vi "Main.vi"(8 "error in (no error)":errorcluster, 11 "StageSPIMBase in":refnum<class "StageSPIM.lvclass">) -> (0 "error out":errorcluster, 3 "component":refnum<class "StageSPIM.lvclass">)   [LabVIEW 2012, in "StageSPIM.lvclass"]
doc: "Main VI of the component."
uses:
  StageSPIM.lvclass
  <vilib>/Distrio/Murmex/Murmex/command_enum.ctl
  StageSPIM.lvclass/StageSPIM.ctl
  <vilib>/Distrio/Murmex/InitialiseMessage/InitialiseMessage.lvclass
  <vilib>/Distrio/Murmex/GenericMessage/GenericMessage.lvclass
  <vilib>/Distrio/Murmex/TerminateMessage/TerminateMessage.lvclass
  <vilib>/Distrio/Murmex/Murmex/update_cluster.ctl
  <vilib>/Distrio/Murmex/StopMessage/StopMessage.lvclass
  <vilib>/Distrio/Murmex/ConfigureMessage/ConfigureMessage.lvclass
  <vilib>/Distrio/Murmex/Murmex/Set configure at initialise.vi
  <vilib>/Distrio/Murmex/Murmex/Set log reference.vi
  <vilib>/Distrio/Murmex/Murmex/Set VI reference.vi
  <vilib>/Distrio/Murmex/Murmex/Get ID.vi
  <vilib>/Distrio/Murmex/Murmex/Set write log to disk.vi
  <vilib>/Distrio/Murmex/Murmex/Murmex.lvclass
  <vilib>/Distrio/Murmex/Message/Message.lvclass
panel:
  in  "Log position?":bool
  in  "button::stop":bool
  in  "button::configure":bool
  in  "button::quit":bool
  in  "Tab Control":enum32{"Main", "Debug"}(tab)
  in  "forwardFocus":bool
  in  "backFocus":bool
  in  "stepFocus":dbl[unit]
  out "currentFocus":dbl[unit]
  in  "speedFocus":dbl[unit]
  in  "targetFocus":dbl[unit]
  in  "forwardY":bool
  in  "backY":bool
  in  "stepY":dbl[unit]
  in  "forwardZ":bool
  in  "backZ":bool
  in  "stepZ":dbl[unit]
  in  "forwardX":bool
  in  "backX":bool
  in  "stepX":dbl[unit]
  in  "forwardA":bool
  in  "backA":bool
  in  "stepA":dbl[unit]
  out "currentA":dbl[unit]
  out "currentX":dbl[unit]
  out "currentY":dbl[unit]
  out "currentZ":dbl[unit]
  in  "speedZ":dbl[unit]
  in  "speedY":dbl[unit]
  in  "speedX":dbl[unit]
  in  "speedA":dbl[unit]
  in  "targetA":dbl[unit]
  in  "targetX":dbl[unit]
  in  "targetY":dbl[unit]
  in  "targetZ":dbl[unit]
  in  "button::send":bool
  out "log":string
  in  "command":T1
  in  "Generic command":string
  in  "ID":string="stage"
  out "terminate?":bool=TRUE
  # "Current\nposition"
  # "Target\nposition"
  # "Steps"
  # "Speed"
  # "A"
  # "X"
  # "Y"
  # "Z"
  # "Focus"
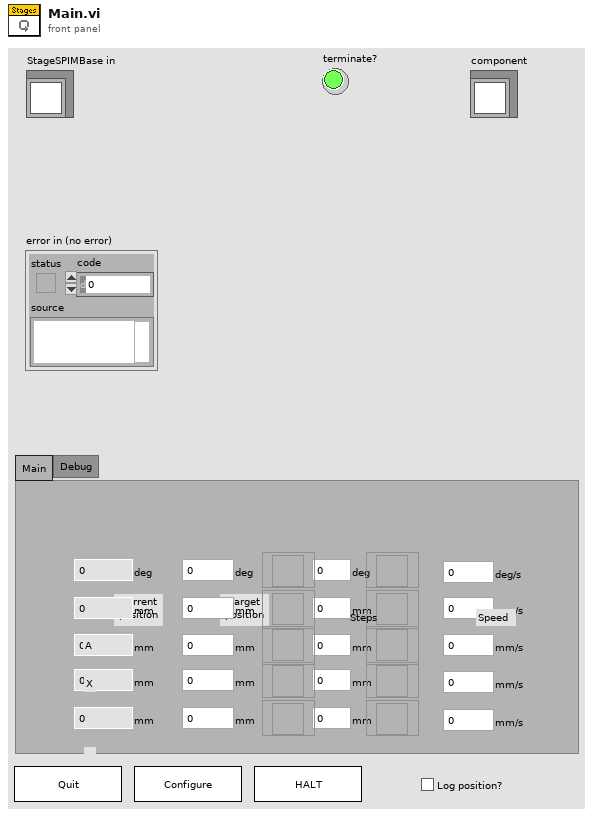
[diagram p1: front panel]
types:
  T1 = typedef "Murmex.lvlib/Murmex.lvclass/command_enum.ctl" = enum16{"null", "initialise", "reset", "terminate", "acknowledge", "update", "inspect", "inform", "proceed", "start", "stop", "fetch", "configure", "generic"}
  T2 = enum8{"Enabled", "Disabled", "Disabled and Grayed Out"}
  T3 = typedef "Murmex.lvlib/Murmex.lvclass/update_cluster.ctl" = cluster{"target ID":string, "key chains":string[], "values":variant[]}
  T4 = typedef "Murmex.lvlib/Murmex.lvclass/Event type enumerations.ctl" = enum16{"before", "after"}
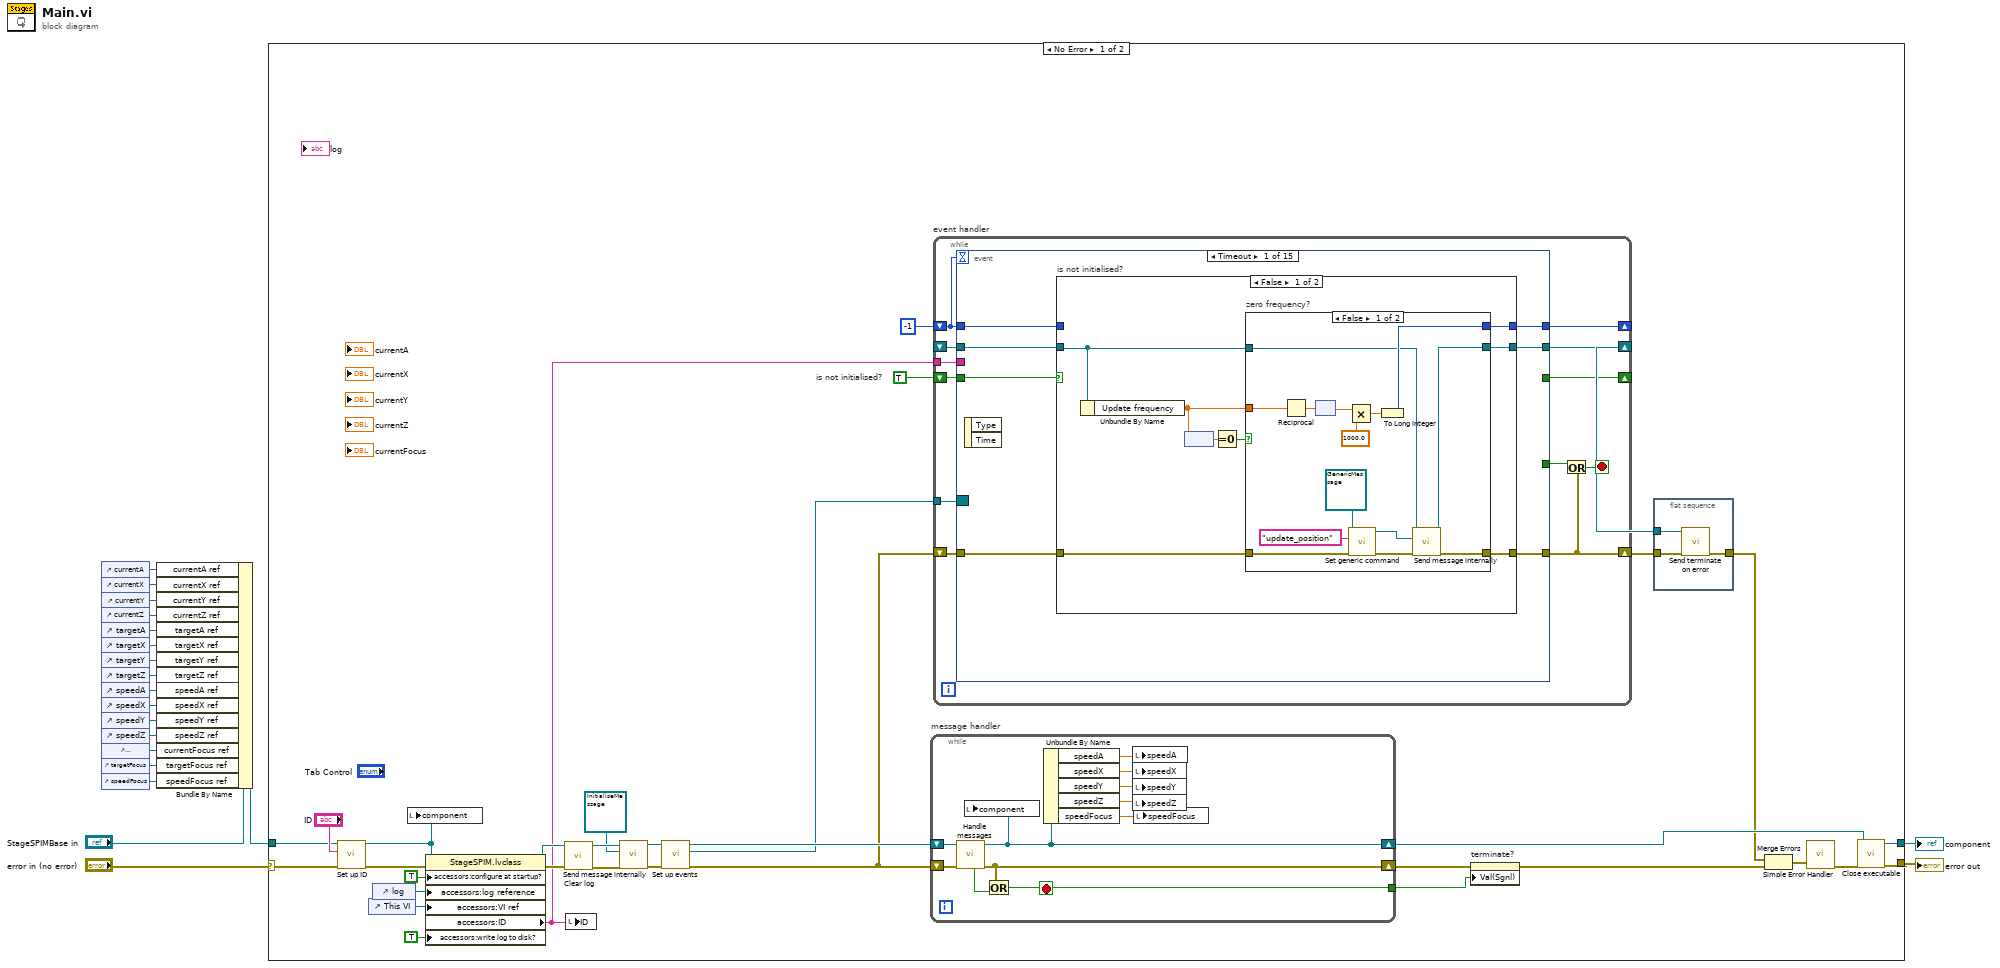
[diagram p0: block diagram]
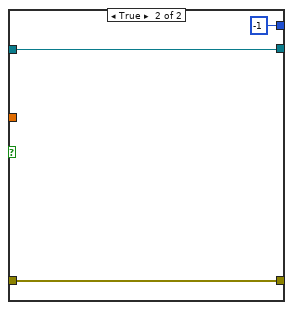
[diagram p2: hidden frame]
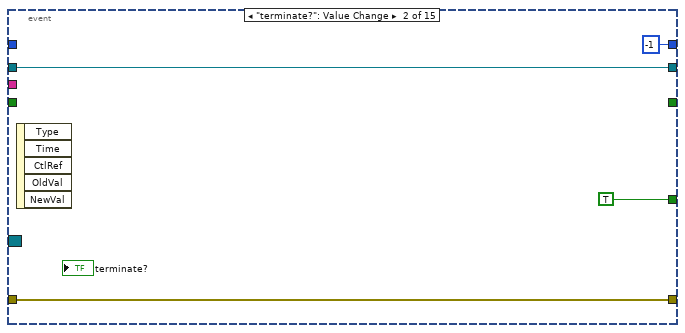
[diagram p4: hidden frame]
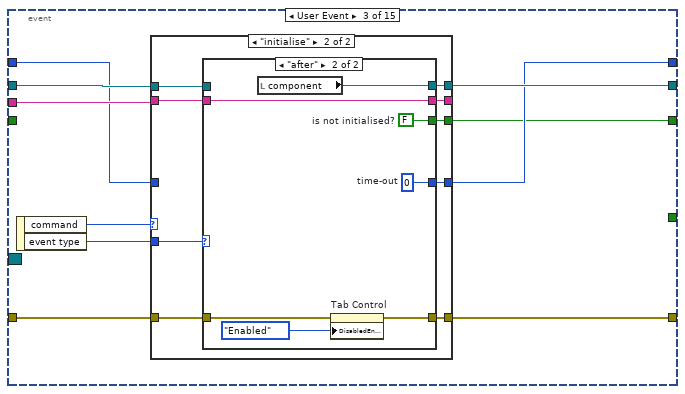
[diagram p5: hidden frame]
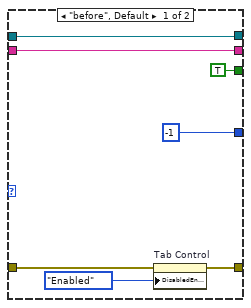
[diagram p7: hidden frame]
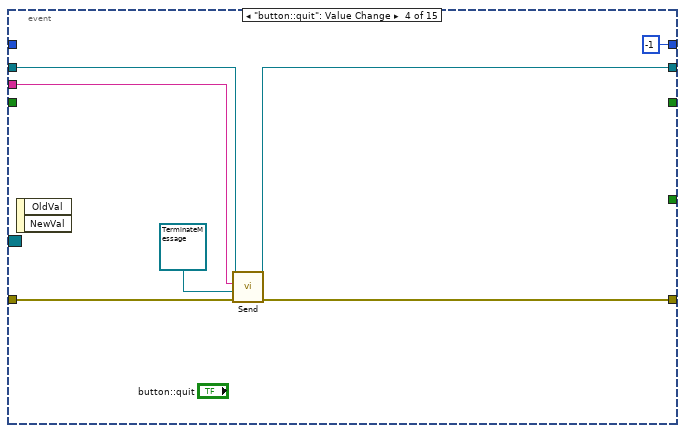
[diagram p8: hidden frame]
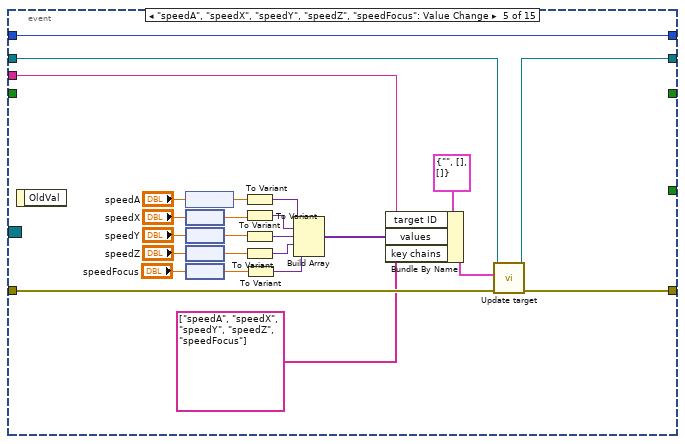
[diagram p9: hidden frame]
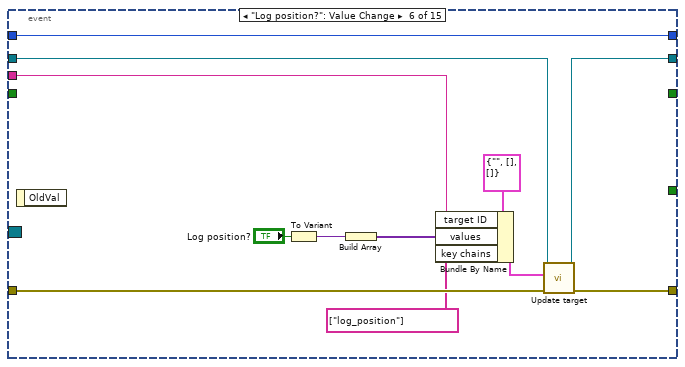
[diagram p10: hidden frame]
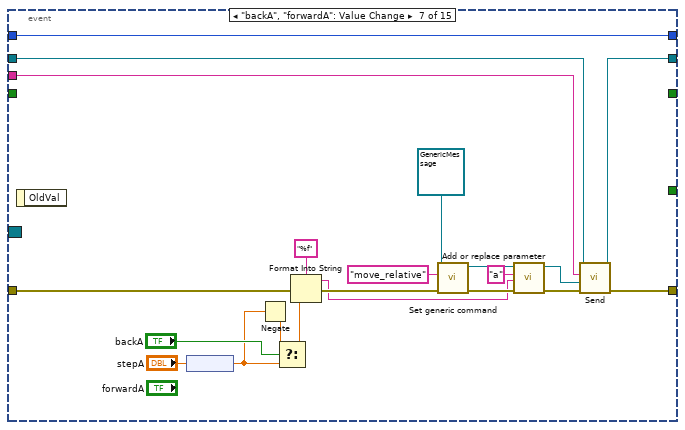
[diagram p11: hidden frame]
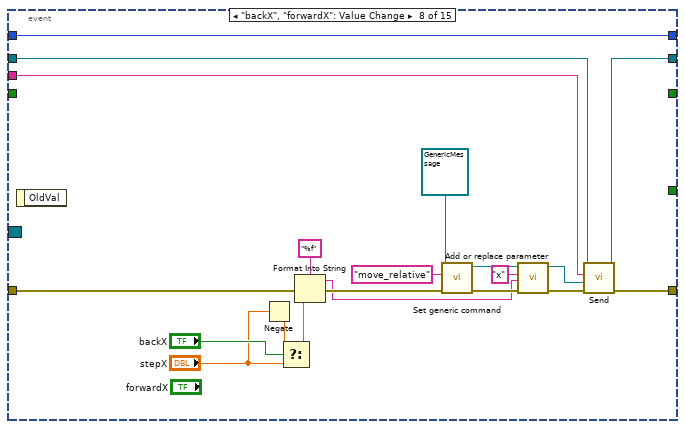
[diagram p12: hidden frame]
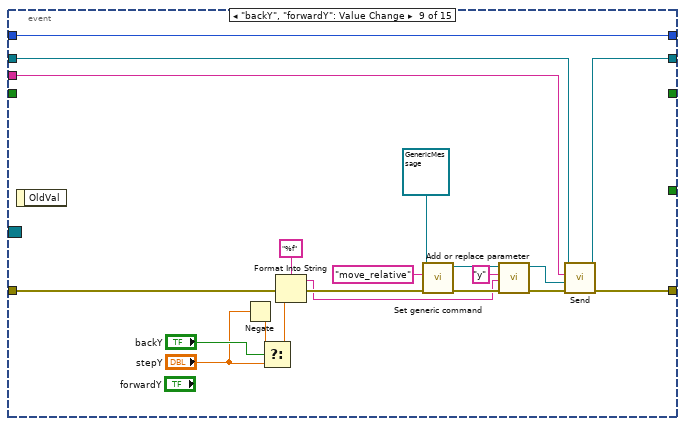
[diagram p13: hidden frame]
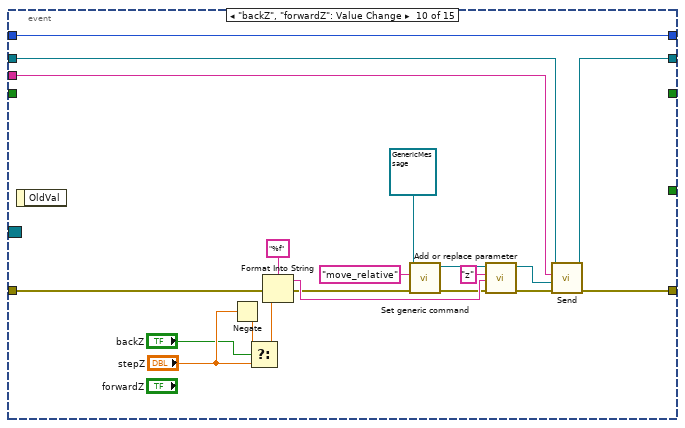
[diagram p14: hidden frame]
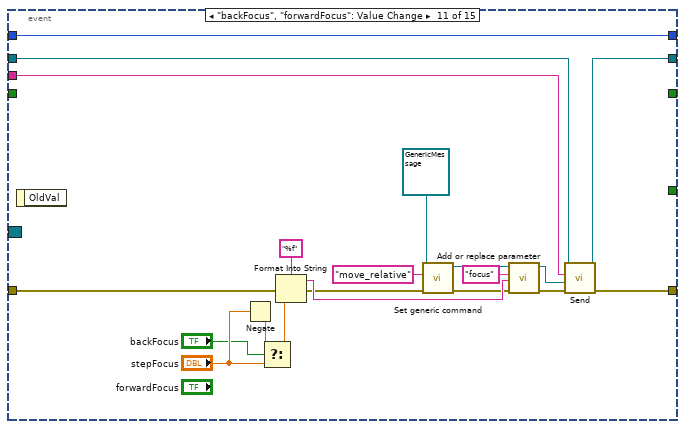
[diagram p15: hidden frame]
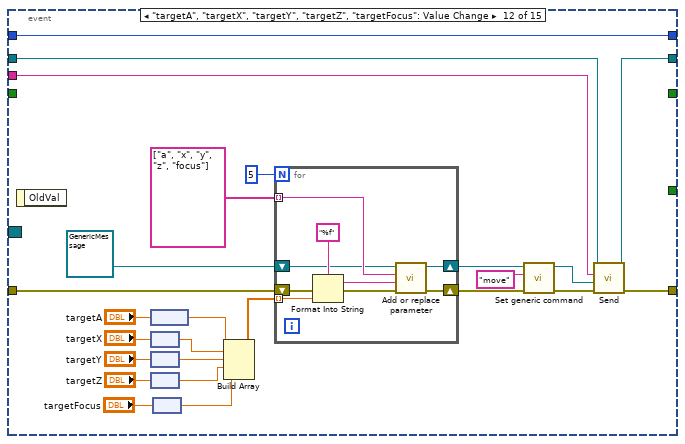
[diagram p16: hidden frame]
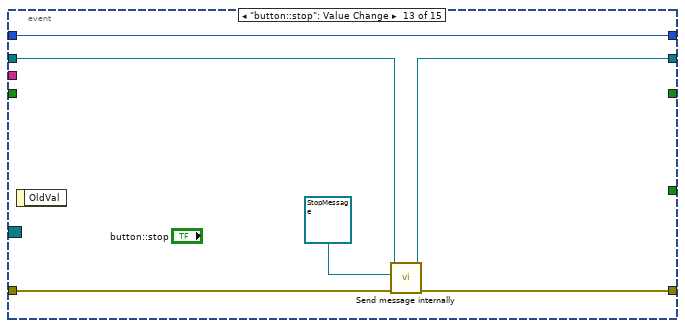
[diagram p17: hidden frame]
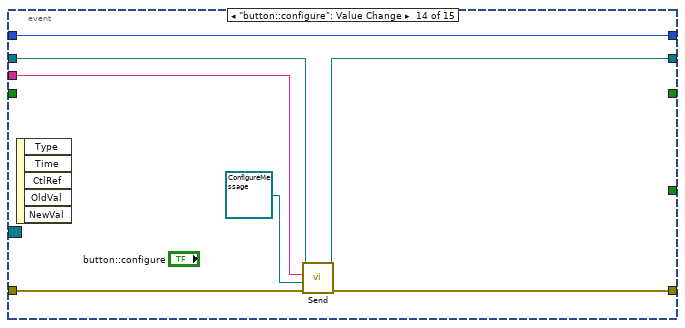
[diagram p18: hidden frame]
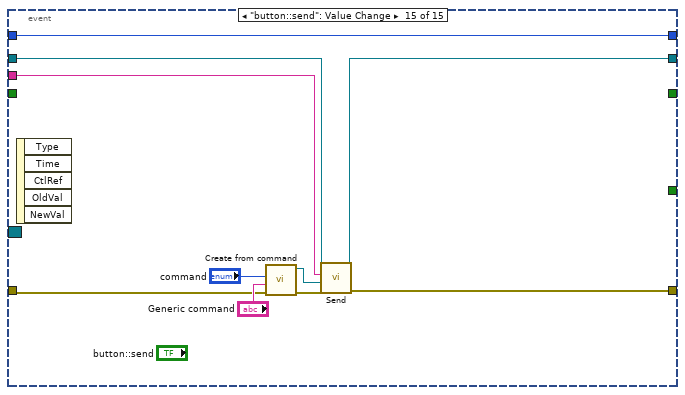
[diagram p19: hidden frame]
diagram:
  n1 = control-ref of="currentA"() -> (w15:refnum<vi>)
  n2 = control-ref of="currentX"() -> (w14:refnum<vi>)
  n3 = control-ref of="currentY"() -> (w13:refnum<vi>)
  n4 = control-ref of="currentZ"() -> (w12:refnum<vi>)
  n5 = control-ref of="targetA"() -> (w11:refnum<vi>)
  n6 = control-ref of="targetX"() -> (w10:refnum<vi>)
  n7 = control-ref of="targetY"() -> (w9:refnum<vi>)
  n8 = control-ref of="targetZ"() -> (w8:refnum<vi>)
  n9 = control-ref of="speedA"() -> (w7:refnum<vi>)
  n10 = control-ref of="speedX"() -> (w6:refnum<vi>)
  n11 = control-ref of="speedY"() -> (w5:refnum<vi>)
  n12 = control-ref of="speedZ"() -> (w4:refnum<vi>)
  n13 = control-ref of="currentFocus"() -> (w3:refnum<vi>)
  n14 = control-ref of="targetFocus"() -> (w2:refnum<vi>)
  n15 = control-ref of="speedFocus"() -> (w1:refnum<vi>)
  n16 = Bundle By Name(cluster="StageSPIMBase in", "currentA ref"=w15, "currentX ref"=w14, "currentY ref"=w13, "currentZ ref"=w12, "targetA ref"=w11, "targetX ref"=w10, "targetY ref"=w9, "targetZ ref"=w8, "speedA ref"=w7, "speedX ref"=w6, "speedY ref"=w5, "speedZ ref"=w4, "currentFocus ref"=w3, "targetFocus ref"=w2, "speedFocus ref"=w1) -> (w18:refnum<class "StageSPIM.lvclass">)
  n17 = case shown="No Error" "error in (no error)" {
    selector: "error in (no error)" -> [w52 w358]
    tunnel: w18 -> [w51 w359]
    tunnel: [w36 w358] -> w17
    tunnel: [w34 w359] -> w16
    frame No Error {
      w26 = TRUE  # is not initialised?
      n18 = call <vilib>:"Set up ID.vi"("error in (no error)"=w52, "component ID"="ID", "MurmexBase in"=w51) -> ("error out"=w50:errorcluster, "MurmexBase out"=w27:refnum<class "StageSPIM.lvclass">)  [unwired: 6 in, 1 out]
      n19 = control-ref of="This VI"() -> (w47:refnum<vi>)
      n20 = control-ref of="log"() -> (w48:refnum<vi>)
      n21 = local write "component"(w27) -> ()
      n22 = property class="StageSPIM.lvclass"(reference=w27, error in=w50, "accessors:configure at startup?"=TRUE ("configure at startup?"), "accessors:log reference"=w48, "accessors:VI ref"=w47, "accessors:write log to disk?"=TRUE ("write log to disk?")) -> (reference out=w45:refnum<class "StageSPIM.lvclass">, error out=w46:errorcluster, "accessors:ID"=w28:string)
      n23 = call <vilib>:"Clear log.vi"("error in (no error)"=w46, "MurmexBase in"=w45) -> ("error out"=w44:errorcluster, "MurmexBase out"=w43:refnum<class "StageSPIM.lvclass">)  [unwired: 8 in]
      n24 = local write "ID"(w28) -> ()
      n25 = call <vilib>:"Send message internally.vi"("error in (no error)"=w44, "Message"=refnum<class "InitialiseMessage.lvclass"> refnum ("Distrio Murmex 1.1:InitialiseMessage"), "Murmex in"=w43) -> ("error out"=w41:errorcluster, "Murmex out"=w40:refnum<class "StageSPIM.lvclass">)  [unwired: 7 in]
      n26 = call <vilib>:"Set up events.vi"("error in (no error)"=w41, "MurmexBase in"=w40) -> ("error out"=w33:errorcluster, "Event Registration Refnum"=w32:refnum<event-registration>, "MurmexBase out"=w39:refnum<class "StageSPIM.lvclass">)  [unwired: 7 in]
      n27 = while "message handler" {
        shift-right: [w355] -> w25
        shift-left: w33 -> [w357]
        shift-right: [w352] -> w35
        shift-left: w39 -> [w356]
        tunnel: [w353] -> w23
        stop <- w353 stop-if-true
        n28 = call <vilib>:"Handle messages.vi"("error in (no error)"=w357, "Murmex in"=w356) -> ("error out"=w355:errorcluster, "Murmex out"=w352:refnum<class "StageSPIM.lvclass">, "terminated?"=w354:bool)  [unwired: 7 in]
        n29 = local write "component"(w352) -> ()
        n30 = Or(x=w355, y=w354) -> (x .or. y?=w353:bool)
        n31 = Unbundle By Name(w352) -> ("speedA"=w351:dbl[unit], "speedX"=w350:dbl[unit], "speedY"=w349:dbl[unit], "speedZ"=w348:dbl[unit], "speedFocus"=w347:dbl[unit])
        n32 = local write "speedA"(w351) -> ()
        n33 = local write "speedX"(w350) -> ()
        n34 = local write "speedY"(w349) -> ()
        n35 = local write "speedZ"(w348) -> ()
        n36 = local write "speedFocus"(w347) -> ()
      }
      n37 = while "event handler" {
        shift-right: [w59] -> w30
        shift-left: w33 -> [w68]
        tunnel: w32 -> [w67]
        shift-right: [w65] -> _
        shift-left: -1 -> [w66]
        shift-right: [w62] -> w22
        shift-left: _ -> [w61]
        shift-right: [w57] -> _
        shift-left: w26 -> [w58]
        tunnel: w28 -> [w63]
        stop <- w64 stop-if-true
        n38 = event shown="[0] Timeout" {
          selector: w67 -> [_ _ _ _ _ _ _ _ _ _ _ _ _ _ _]
          dyn-events: _ -> [_ _ _ _ _ _ _ _ _ _ _ _ _ _ _]
          timeout: w66 -> [_ _ _ _ _ _ _ _ _ _ _ _ _ _ _]
          tunnel: w68 -> [w74 w107 w117 w150 w175 w185 w208 w211 w233 w253 w274 w293 w329 w336 w342]
          tunnel: w66 -> [w69 _ w109 _ w160 w182 w209 w210 w232 w254 w270 w309 w327 w330 w338]
          tunnel: [w75 -1 ("time-out") w110 -1 ("time-out") w160 w182 w209 w210 w232 w254 w270 w309 w327 w330 w338] -> w65
          tunnel: [w73 w107 w111 w149 w174 w186 w198 w217 w237 w256 w277 w313 w325 w335 w341] -> w59
          tunnel: w63 -> [_ _ w114 w146 w173 w181 w195 w214 w234 w255 w271 w310 _ w333 w337]
          tunnel: w61 -> [w71 w105 w113 w148 w172 w184 w197 w215 w235 w250 w273 w311 w328 w332 w340]
          tunnel: [w72 w105 w112 w147 w171 w183 w196 w216 w236 w257 w272 w312 w326 w331 w339] -> w62
          tunnel: [_ TRUE _ _ _ _ _ _ _ _ _ _ _ _ _] -> w60
          tunnel: w58 -> [w70 _ _ _ _ _ _ _ _ _ _ _ _ _ _]
          tunnel: [_ _ w108 _ _ _ _ _ _ _ _ _ _ _ _] -> w57
          event Timeout {
            n39 = event-data() -> ()  [unwired: 1 in, 2 out]
            n40 = case "is not initialised?" shown="False" w70 {
              tunnel: [w83 w101] -> w75
              tunnel: w74 -> [w82 w103]
              tunnel: [w81 w103] -> w73
              tunnel: [w80 w102] -> w72
              tunnel: w71 -> [w76 w102]
              tunnel: w69 -> [_ w101]
              frame False {
                n41 = Unbundle By Name(w76) -> ("Update frequency"=w79:dbl[unit])
                n42 = node(w79) -> (w78:dbl)
                n43 = Equal To 0?(x=w78) -> (x = 0?=w77:bool)
                n44 = case "zero frequency?" shown="False" w77 {
                  tunnel: [w93 -1] -> w83
                  tunnel: w82 -> [w85 w99]
                  tunnel: [w86 w99] -> w81
                  tunnel: w76 -> [w91 w100]
                  tunnel: [w84 w100] -> w80
                  tunnel: w79 -> [w92 _]
                  frame False {
                    n45 = Reciprocal(x=w92) -> (1/x=w97:dbl[unit])
                    n46 = node(w97) -> (w95:dbl)
                    n47 = Multiply(x=w95, y=1000.0) -> (x*y=w94:dbl)
                    n48 = call <vilib>:"Set generic command.vi"("error in (no error)"=w85, "generic command"="update_position", "GenericMessage in"=refnum<class "GenericMessage.lvclass"> refnum ("Message in")) -> ("error out"=w87:errorcluster, "GenericMessage out"=w88:refnum<class "GenericMessage.lvclass">)  [unwired: 7 in]
                    n49 = To Long Integer(number=w94) -> (32bit integer=w93:i32)
                    n50 = call <vilib>:"Send message internally.vi"("error in (no error)"=w87, "Message"=w88, "Murmex in"=w91) -> ("error out"=w86:errorcluster, "Murmex out"=w84:refnum<class "StageSPIM.lvclass">)  [unwired: 7 in]
                  }
                  frame True {
                  }
                }
              }
              frame True {
              }
            }
          }
          event "terminate?": Value Change {
            n51 = event-data() -> ()  [unwired: 1 in, 5 out]
          }
          event User Event {
            n52 = event-data() -> ("command"=w116:T1, "event type"=w115:T4)  [unwired: 1 in]
            n53 = case shown="\"initialise\"" w116 {
              tunnel: w117 -> [w119 w130]
              tunnel: [w119 w129] -> w111
              tunnel: w114 -> [w121 w128]
              tunnel: [w120 w127] -> w112
              tunnel: w113 -> [w120 w126]
              tunnel: [w121 w125] -> _
              tunnel: w115 -> [_ w124]
              tunnel: [w118 w123] -> w110
              tunnel: w109 -> [w118 _]
              tunnel: [_ w122] -> w108
              frame "null", Default {
              }
              frame "initialise" {
                n54 = case shown="\"after\"" w124 {
                  tunnel: [w136 w143] -> w129
                  tunnel: w130 -> [w137 w144]
                  tunnel: w128 -> [w134 w140]
                  tunnel: [w133 w142] -> w127
                  tunnel: w126 -> [w133 _]
                  tunnel: [w134 w140] -> w125
                  tunnel: [-1 w139] -> w123
                  tunnel: [TRUE ("is not initialised?") w138] -> w122
                  frame "before", Default {
                    n55 = property on="Tab Control" class="TabCtl (strict)"(error in=w137, "DisabledEnum"=T2."Enabled" ("Disabled")) -> (error out=w136:errorcluster)  [unwired: 1 in, 1 out]
                  }
                  frame "after" {
                    w138 = FALSE  # is not initialised?
                    w139 = 0  # time-out
                    n56 = local read "component"() -> (w142:refnum<class "StageSPIM.lvclass">)
                    n57 = property on="Tab Control" class="TabCtl (strict)"(error in=w144, "DisabledEnum"=T2."Enabled" ("Disabled")) -> (error out=w143:errorcluster)  [unwired: 1 in, 1 out]
                  }
                }
              }
            }
          }
          event "button::quit": Value Change {
            n58 = event-data() -> ()  [unwired: 1 in, 2 out]
            n59 = call <vilib>:"Send.vi"("error in (no error)"=w150, "Message"=refnum<class "TerminateMessage.lvclass"> refnum ("Murmex.lvlib:TerminateMessage"), "recipient"=w146, "Murmex in"=w148) -> ("error out"=w149:errorcluster, "Murmex out"=w147:refnum<class "StageSPIM.lvclass">)  [unwired: 6 in]
          }
          event "speedA", "speedX", "speedY", "speedZ", "speedFocus": Value Change {
            n60 = event-data() -> ()  [unwired: 1 in, 1 out]
            n61 = node("speedA") -> (w159:dbl)
            n62 = node("speedX") -> (w156:dbl)
            n63 = node("speedY") -> (w157:dbl)
            n64 = node("speedZ") -> (w158:dbl)
            n65 = node("speedFocus") -> (w154:dbl)
            n66 = To Variant(anything=w159) -> (Variant=w166:variant)
            n67 = To Variant(anything=w156) -> (Variant=w165:variant)
            n68 = To Variant(anything=w157) -> (Variant=w164:variant)
            n69 = To Variant(anything=w158) -> (Variant=w163:variant)
            n70 = To Variant(anything=w154) -> (Variant=w153:variant)
            n71 = Build Array(w166, w165, w164, w163, w153) -> (w162:variant[])
            n72 = Bundle By Name(cluster=T3 {"target ID"="", "key chains"=[], "values"=[]} ("update cluster"), "target ID"=w173, "values"=w162, "key chains"=string[] ["speedA", "speedX", "speedY", "speedZ", "speedFocus"]) -> (w152:T3)
            n73 = call <vilib>:"Update target.vi"("error in (no error)"=w175, "update cluster"=w152, "MurmexBase in"=w172) -> ("error out"=w174:errorcluster, "MurmexBase out"=w171:refnum<class "StageSPIM.lvclass">)  [unwired: 7 in]
          }
          event "Log position?": Value Change {
            n74 = event-data() -> ()  [unwired: 1 in, 1 out]
            n75 = To Variant(anything="Log position?") -> (Variant=w179:variant)
            n76 = Build Array(w179) -> (w178:variant[])
            n77 = Bundle By Name(cluster=T3 {"target ID"="", "key chains"=[], "values"=[]} ("update cluster"), "target ID"=w181, "values"=w178, "key chains"=string[] ["log_position"]) -> (w187:T3)
            n78 = call <vilib>:"Update target.vi"("error in (no error)"=w185, "update cluster"=w187, "MurmexBase in"=w184) -> ("error out"=w186:errorcluster, "MurmexBase out"=w183:refnum<class "StageSPIM.lvclass">)  [unwired: 7 in]
          }
          event "backA", "forwardA": Value Change {
            n79 = event-data() -> ()  [unwired: 1 in, 1 out]
            n80 = node("stepA") -> (w189:dbl)
            n81 = Negate(x=w189) -> (-x=w202:dbl)
            n82 = Select(t=w202, s="backA", f=w189) -> (s? t:f=w191:dbl)
            n83 = Format Into String(format string="%f", error in=w208, w191) -> (resulting string=w192:string, error out=w199:errorcluster)  [unwired: 1 in]
            n84 = call <vilib>:"Set generic command.vi"("error in (no error)"=w199, "generic command"="move_relative", "GenericMessage in"=refnum<class "GenericMessage.lvclass"> refnum ("Distrio Murmex 1.1:GenericMessage")) -> ("error out"=w206:errorcluster, "GenericMessage out"=w204:refnum<class "GenericMessage.lvclass">)  [unwired: 7 in]
            n85 = call <vilib>:"Add or replace parameter.vi"("error in (no error)"=w206, "value"=w192, "name"="a", "Message in"=w204) -> ("error out"=w205:errorcluster, "Message out"=w193:refnum<class "GenericMessage.lvclass">)  [unwired: 6 in]
            n86 = call <vilib>:"Send.vi"("error in (no error)"=w205, "Message"=w193, "recipient"=w195, "Murmex in"=w197) -> ("error out"=w198:errorcluster, "Murmex out"=w196:refnum<class "StageSPIM.lvclass">)  [unwired: 6 in]
          }
          event "backX", "forwardX": Value Change {
            n87 = event-data() -> ()  [unwired: 1 in, 1 out]
            n88 = Negate(x="stepX") -> (-x=w224:dbl[unit])
            n89 = Select(t=w224, s="backX", f="stepX") -> (s? t:f=w219:dbl[unit])
            n90 = Format Into String(format string="%f", error in=w211, w219) -> (resulting string=w220:string, error out=w223:errorcluster)  [unwired: 1 in]
            n91 = call <vilib>:"Set generic command.vi"("error in (no error)"=w223, "generic command"="move_relative", "GenericMessage in"=refnum<class "GenericMessage.lvclass"> refnum ("Distrio Murmex 1.1:GenericMessage")) -> ("error out"=w228:errorcluster, "GenericMessage out"=w226:refnum<class "GenericMessage.lvclass">)  [unwired: 7 in]
            n92 = call <vilib>:"Add or replace parameter.vi"("error in (no error)"=w228, "value"=w220, "name"="x", "Message in"=w226) -> ("error out"=w227:errorcluster, "Message out"=w221:refnum<class "GenericMessage.lvclass">)  [unwired: 6 in]
            n93 = call <vilib>:"Send.vi"("error in (no error)"=w227, "Message"=w221, "recipient"=w214, "Murmex in"=w215) -> ("error out"=w217:errorcluster, "Murmex out"=w216:refnum<class "StageSPIM.lvclass">)  [unwired: 6 in]
          }
          event "backY", "forwardY": Value Change {
            n94 = event-data() -> ()  [unwired: 1 in, 1 out]
            n95 = Negate(x="stepY") -> (-x=w244:dbl[unit])
            n96 = Select(t=w244, s="backY", f="stepY") -> (s? t:f=w239:dbl[unit])
            n97 = Format Into String(format string="%f", error in=w233, w239) -> (resulting string=w240:string, error out=w243:errorcluster)  [unwired: 1 in]
            n98 = call <vilib>:"Set generic command.vi"("error in (no error)"=w243, "generic command"="move_relative", "GenericMessage in"=refnum<class "GenericMessage.lvclass"> refnum ("Distrio Murmex 1.1:GenericMessage")) -> ("error out"=w248:errorcluster, "GenericMessage out"=w246:refnum<class "GenericMessage.lvclass">)  [unwired: 7 in]
            n99 = call <vilib>:"Add or replace parameter.vi"("error in (no error)"=w248, "value"=w240, "name"="y", "Message in"=w246) -> ("error out"=w247:errorcluster, "Message out"=w241:refnum<class "GenericMessage.lvclass">)  [unwired: 6 in]
            n100 = call <vilib>:"Send.vi"("error in (no error)"=w247, "Message"=w241, "recipient"=w234, "Murmex in"=w235) -> ("error out"=w237:errorcluster, "Murmex out"=w236:refnum<class "StageSPIM.lvclass">)  [unwired: 6 in]
          }
          event "backZ", "forwardZ": Value Change {
            n101 = event-data() -> ()  [unwired: 1 in, 1 out]
            n102 = Negate(x="stepZ") -> (-x=w263:dbl[unit])
            n103 = Select(t=w263, s="backZ", f="stepZ") -> (s? t:f=w268:dbl[unit])
            n104 = Format Into String(format string="%f", error in=w253, w268) -> (resulting string=w267:string, error out=w264:errorcluster)  [unwired: 1 in]
            n105 = call <vilib>:"Set generic command.vi"("error in (no error)"=w264, "generic command"="move_relative", "GenericMessage in"=refnum<class "GenericMessage.lvclass"> refnum ("Distrio Murmex 1.1:GenericMessage")) -> ("error out"=w259:errorcluster, "GenericMessage out"=w261:refnum<class "GenericMessage.lvclass">)  [unwired: 7 in]
            n106 = call <vilib>:"Add or replace parameter.vi"("error in (no error)"=w259, "value"=w267, "name"="z", "Message in"=w261) -> ("error out"=w260:errorcluster, "Message out"=w266:refnum<class "GenericMessage.lvclass">)  [unwired: 6 in]
            n107 = call <vilib>:"Send.vi"("error in (no error)"=w260, "Message"=w266, "recipient"=w255, "Murmex in"=w250) -> ("error out"=w256:errorcluster, "Murmex out"=w257:refnum<class "StageSPIM.lvclass">)  [unwired: 6 in]
          }
          event "backFocus", "forwardFocus": Value Change {
            n108 = event-data() -> ()  [unwired: 1 in, 1 out]
            n109 = Negate(x="stepFocus") -> (-x=w283:dbl[unit])
            n110 = Select(t=w283, s="backFocus", f="stepFocus") -> (s? t:f=w288:dbl[unit])
            n111 = Format Into String(format string="%f", error in=w274, w288) -> (resulting string=w287:string, error out=w284:errorcluster)  [unwired: 1 in]
            n112 = call <vilib>:"Set generic command.vi"("error in (no error)"=w284, "generic command"="move_relative", "GenericMessage in"=refnum<class "GenericMessage.lvclass"> refnum ("Distrio Murmex 1.1:GenericMessage")) -> ("error out"=w279:errorcluster, "GenericMessage out"=w281:refnum<class "GenericMessage.lvclass">)  [unwired: 7 in]
            n113 = call <vilib>:"Add or replace parameter.vi"("error in (no error)"=w279, "value"=w287, "name"="focus", "Message in"=w281) -> ("error out"=w280:errorcluster, "Message out"=w286:refnum<class "GenericMessage.lvclass">)  [unwired: 6 in]
            n114 = call <vilib>:"Send.vi"("error in (no error)"=w280, "Message"=w286, "recipient"=w271, "Murmex in"=w273) -> ("error out"=w277:errorcluster, "Murmex out"=w272:refnum<class "StageSPIM.lvclass">)  [unwired: 6 in]
          }
          event "targetA", "targetX", "targetY", "targetZ", "targetFocus": Value Change {
            n115 = event-data() -> ()  [unwired: 1 in, 1 out]
            n116 = node("targetA") -> (w296:dbl)
            n117 = node("targetX") -> (w300:dbl)
            n118 = node("targetY") -> (w297:dbl)
            n119 = node("targetZ") -> (w292:dbl)
            n120 = node("targetFocus") -> (w290:dbl)
            n121 = Build Array(w296, w300, w297, w292, w290) -> (w294:dbl[])
            n122 = for {
              N: 5 -> [_]
              shift-right: [w321] -> w306
              shift-left: w293 -> [w320]
              tunnel: string[] ["a", "x", "y", "z", "focus"] -> [w319] mode=indexing
              shift-right: [w317] -> w302
              shift-left: refnum<class "GenericMessage.lvclass"> refnum ("Distrio Murmex 1.1:GenericMessage") -> [w318]
              tunnel: w294 -> [w316] mode=indexing
              n123 = Format Into String(format string="%f", error in=w320, w316) -> (resulting string=w315:string, error out=w322:errorcluster)  [unwired: 1 in]
              n124 = call <vilib>:"Add or replace parameter.vi"("error in (no error)"=w322, "value"=w315, "name"=w319, "Message in"=w318) -> ("error out"=w321:errorcluster, "Message out"=w317:refnum<class "GenericMessage.lvclass">)  [unwired: 6 in]
            }
            n125 = call <vilib>:"Set generic command.vi"("error in (no error)"=w306, "generic command"="move", "GenericMessage in"=w302) -> ("error out"=w308:errorcluster, "GenericMessage out"=w307:refnum<class "GenericMessage.lvclass">)  [unwired: 7 in]
            n126 = call <vilib>:"Send.vi"("error in (no error)"=w308, "Message"=w307, "recipient"=w310, "Murmex in"=w311) -> ("error out"=w313:errorcluster, "Murmex out"=w312:refnum<class "StageSPIM.lvclass">)  [unwired: 6 in]
          }
          event "button::stop": Value Change {
            n127 = event-data() -> ()  [unwired: 1 in, 1 out]
            n128 = call <vilib>:"Send message internally.vi"("error in (no error)"=w329, "Message"=refnum<class "StopMessage.lvclass"> refnum ("Distrio Murmex 1.5:StopMessage"), "Murmex in"=w328) -> ("error out"=w325:errorcluster, "Murmex out"=w326:refnum<class "StageSPIM.lvclass">)  [unwired: 7 in]
          }
          event "button::configure": Value Change {
            n129 = event-data() -> ()  [unwired: 1 in, 5 out]
            n130 = call <vilib>:"Send.vi"("error in (no error)"=w336, "Message"=refnum<class "ConfigureMessage.lvclass"> refnum ("Distrio Murmex 1.1:ConfigureMessage"), "recipient"=w333, "Murmex in"=w332) -> ("error out"=w335:errorcluster, "Murmex out"=w331:refnum<class "StageSPIM.lvclass">)  [unwired: 6 in]
          }
          event "button::send": Value Change {
            n131 = event-data() -> ()  [unwired: 1 in, 5 out]
            n132 = call <vilib>:"Create from command.vi"("error in (no error)"=w342, "generic command"="Generic command", "command"="command") -> ("error out"=w344:errorcluster, "Message out"=w345:refnum<class "Message.lvclass">)  [unwired: 7 in]
            n133 = call <vilib>:"Send.vi"("error in (no error)"=w344, "Message"=w345, "recipient"=w337, "Murmex in"=w340) -> ("error out"=w341:errorcluster, "Murmex out"=w339:refnum<class "StageSPIM.lvclass">)  [unwired: 6 in]
          }
        }
        n134 = Or(x=w60, y=w59) -> (x .or. y?=w64:bool)
      }
      n135 = property on="terminate?" class="Bool (strict)"(error in=w25, "Val(Sgnl)"=w23) -> (error out=w24:errorcluster)  [unwired: 1 in, 1 out]
      n136 = flat-sequence {
        tunnel: w30 -> [w56]
        tunnel: [w55] -> w29
        tunnel: w22 -> [w54]
        frame #0 {
          n137 = call <vilib>:"Send terminate on error.vi"("error in (no error)"=w56, "Murmex in"=w54) -> ("error out"=w55:errorcluster)  [unwired: 8 in, 1 out]
        }
      }
      n138 = Merge Errors(w29, w24) -> (w38:errorcluster)
      n139 = call <vilib>:"Simple Error Handler.vi"("error in (no error)"=w38) -> ("error out"=w37:errorcluster)  [unwired: 4 in, 4 out]
      n140 = call <vilib>:"Close executable.vi"("error in (no error)"=w37, "MurmexBase in"=w35) -> ("error out"=w36:errorcluster, "MurmexBase out"=w34:refnum<class "StageSPIM.lvclass">)  [unwired: 8 in]
    }
    frame Error {
    }
  }
  "error out" <- w17
  "component" <- w16
